vi "DeQ_DaQ_QMH.vi"(8 "Error In":errorcluster, 11 "Queue In":refnum<queue>) -> (0 "Error Out":errorcluster, 1 "Message":variant, 2 "Instruction":T1=enum."Start DaQ", 3 "Queue Out":refnum<queue>)   [LabVIEW 2021, in "Queues.lvlib"]
doc: "This subVI is used to dequeue and unbundle the elements of DaQ QMH queue."
uses:
  Queues.lvlib
  Tipski Definicii/QMH_Daq_States.ctl
panel:
  # "Input"
  # "Output"
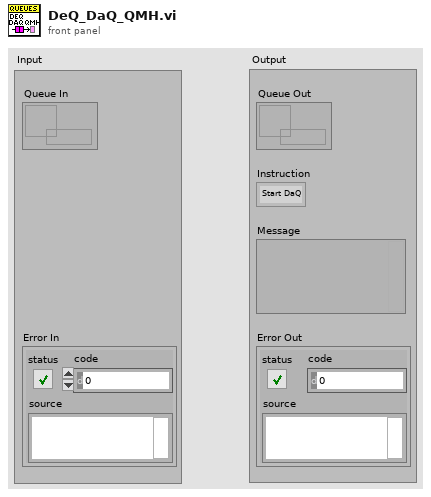
[diagram p1: front panel]
types:
  T1 = typedef "QMH_Daq_States.ctl" = enum16{"Idle", "Start DaQ", "DaQ", "Generate Message", "Stop DaQ", "End"}
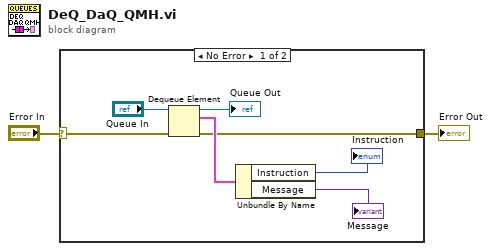
[diagram p0: block diagram]
diagram:
  n1 = case shown="No Error" "Error In" {
    selector: "Error In" -> [w7 w10]
    tunnel: [w6 w10] -> w1
    frame No Error {
      n2 = Dequeue Element(queue="Queue In", error in (no error)=w7) -> (queue out=→"Queue Out":refnum<queue>, element=w9:cluster{"Instruction":T1, "Message":variant}, error out=w6:errorcluster)  [unwired: 1 in, 1 out]
      n3 = Unbundle By Name(w9) -> ("Instruction"=→"Instruction":T1, "Message"=→"Message":variant)
    }
    frame Error {
    }
  }
  "Error Out" <- w1
